vi "DrawScalebar.vi"(0 "CameraController in":refnum<class "CameraController.lvclass">, 5 "Image In":T1, 7 "ScaleBarSize":dbl min=0.0 max=50.0, 9 "Binning":dbl min=0.0 max=50.0, 11 "error in (no error)":errorcluster) -> (4 "CameraController out":refnum<class "CameraController.lvclass">, 6 "Image Out":T1, 15 "error out":errorcluster)   [LabVIEW 2020, in "CameraController.lvlib" / "CameraController.lvclass"]
uses:
  CameraController.lvclass
  <vilib>/vision/Image Controls.llb/IMAQ Image.ctl
  <vilib>/vision/NI_Vision_Development_Module.lvlib
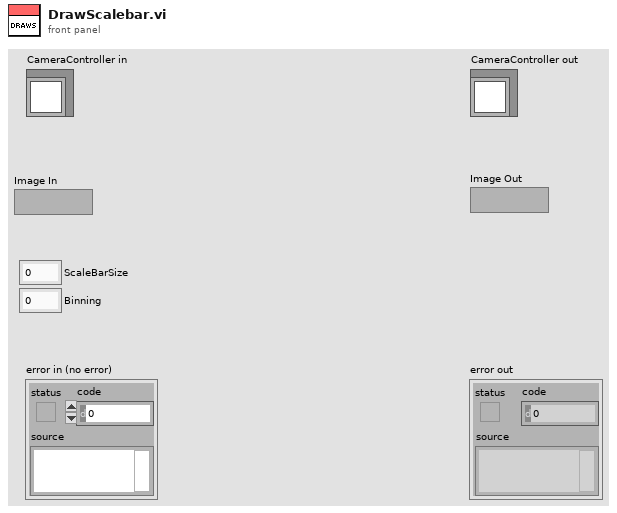
[diagram p1: front panel]
types:
  T1 = typedef "IMAQ Image.ctl" = refnum<image>
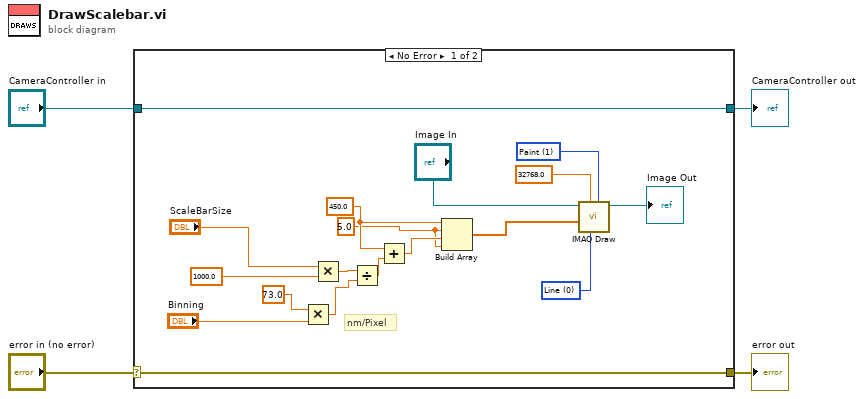
[diagram p0: block diagram]
diagram:
  n1 = case shown="No Error" "error in (no error)" {
    selector: "error in (no error)" -> [w21 w24]
    tunnel: [w21 w24] -> w3
    tunnel: [w22 w23] -> w1
    tunnel: "CameraController in" -> [w22 w23]
    frame No Error {
      w7 = u16 1 items=["Frame", "Paint", "Invert Frame", "Invert Paint"] ("Draw Mode")
      w6 = u16 0 items=["Line", "Rectangle", "Oval"] ("Shape to draw")
      w8 = 5.0 ("element")
      w10 = 450.0 ("element")
      # "nm/Pixel"
      n2 = Multiply(x=73.0 ("y"), y="Binning") -> (x*y=w20:dbl)
      n3 = Multiply(x="ScaleBarSize", y=1000.0) -> (x*y=w14:dbl)
      n4 = Divide(x=w14, y=w20) -> (x/y=w15:dbl)
      n5 = Add(x=w10, y=w15) -> (x+y=w16:dbl)
      n6 = Build Array(w10, w8, w16, w8) -> (w17:dbl[])
      n7 = call "IMAQ Draw"("Draw Mode"=w7, "Shape to draw"=w6, "Pixel Color"=sgl 32768.0, "Coordinates"=w17, "Image Src"="Image In") -> ("Image Dst Out"=→"Image Out":T1)  [unwired: 5 in, 1 out]
    }
    frame Error {
    }
  }
  "error out" <- w3
  "CameraController out" <- w1
